vi "GetEpochTime.vi"(7 "Parameters for Optic stimulation":T1) -> (3 "Epoch begin / end":dbl[][](array[numeric]))   [LabVIEW 2017]
uses:
  Parameters for Optic Stimulation.ctl
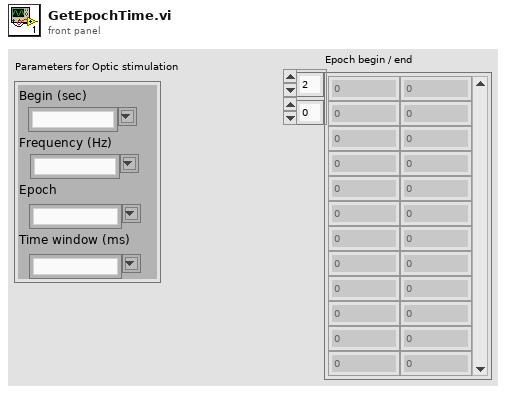
[diagram p1: front panel]
types:
  T1 = typedef "Parameters for Optic Stimulation.ctl" = cluster{"Begin (sec)":string, "Frequency (Hz)":string, "Epoch":string, "Time window (ms)":string}
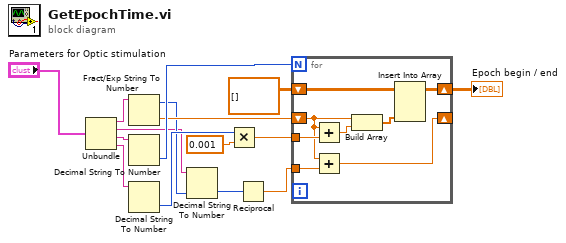
[diagram p0: block diagram]
diagram:
  n1 = Unbundle("Parameters for Optic stimulation") -> ("Begin (sec)"=w12:string, "Frequency (Hz)"=w5:string, "Epoch"=w14:string, "Time window (ms)"=w10:string)
  n2 = Fract/Exp String To Number(string=w12) -> (offset past number=w6:i32, number=w11:dbl)  [unwired: 3 in]
  n3 = Decimal String To Number(string=w14) -> (number=w13:i32)  [unwired: 2 in, 1 out]
  n4 = Decimal String To Number(string=w10) -> (number=w9:i32)  [unwired: 2 in, 1 out]
  n5 = Decimal String To Number(string=w5, default (0L)=w6) -> (number=w4:i32)  [unwired: 1 in, 1 out]
  n6 = Multiply(x=w9, y=0.001) -> (x*y=w7:dbl)
  n7 = Reciprocal(x=w4) -> (1/x=w3:dbl)
  n8 = for {
    N: w13 -> [_]
    tunnel: w7 -> [w18]
    tunnel: w3 -> [w23]
    shift-right: [w21] -> w1
    shift-left: dbl[][] [] -> [w20]
    shift-right: [w19] -> _
    shift-left: w11 -> [w17]
    n9 = Add(x=w17, y=w18) -> (x+y=w16:dbl)
    n10 = Add(x=w17, y=w23) -> (x+y=w19:dbl)
    n11 = Build Array(w17, w16) -> (w22:dbl[])
    n12 = Insert Into Array(array=w20, new element=w22) -> (w21:dbl[][])  [unwired: 2 in]
  }
  "Epoch begin / end" <- w1
